vi "Get DLL version.vi"() -> (0 "Error":errorcluster, 2 "DLL version":string)   [LabVIEW 2014]
uses:
  Program Files (x86)/Coherent/HOPS/CohrHOPS.dll
panel:
  # "PN 04/11/2014"
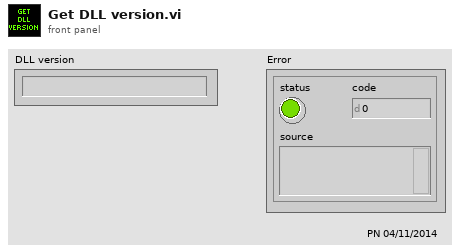
[diagram p1: front panel]
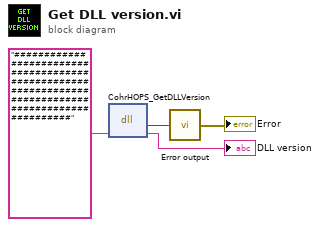
[diagram p0: block diagram]
diagram:
  n1 = dll-call lib="C:/Program Files (x86)/Coherent/HOPS/CohrHOPS.dll" fn="CohrHOPS_GetDLLVersion"("version"="####################################################################################################" ("headType")) -> ("return value"=w3:i32, "version"=→"DLL version":string)  [unwired: 3 in, 2 out]
  n2 = call "Error output.vi"("I32 err code"=w3) -> ("Error Out"=→"Error":errorcluster)
